vi "Move to final location.vi"(8 "error in (no error)":errorcluster, 11 "DAQOrcaFlash in":refnum<class "DAQOrcaFlash.lvclass">) -> (0 "error out":errorcluster, 3 "DAQOrcaFlash out":refnum<class "DAQOrcaFlash.lvclass">)   [LabVIEW 2012, in "DAQOrcaFlash.lvclass"]
uses:
  DAQOrcaFlash.lvclass
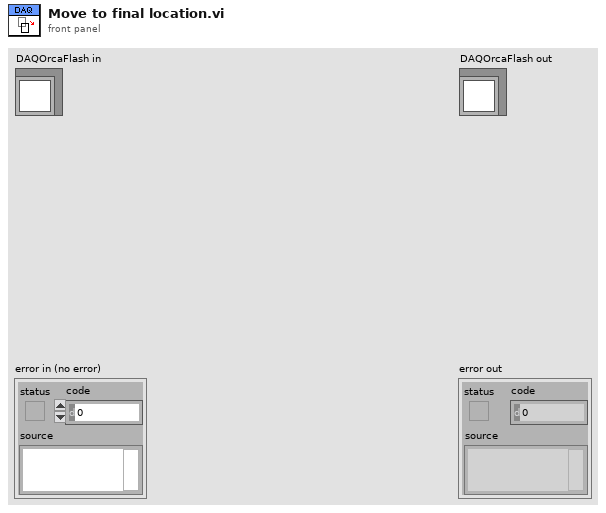
[diagram p1: front panel]
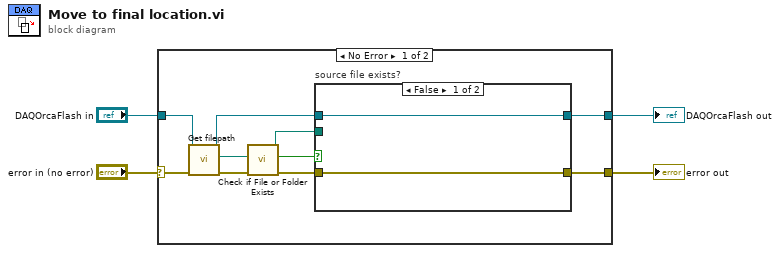
[diagram p0: block diagram]
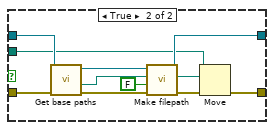
[diagram p2: hidden frame]
diagram:
  n1 = case shown="No Error" "error in (no error)" {
    selector: "error in (no error)" -> [w14 w29]
    tunnel: [w13 w29] -> w3
    tunnel: [w10 w28] -> w1
    tunnel: "DAQOrcaFlash in" -> [w11 w28]
    frame No Error {
      n2 = call "Get filepath.vi"("error in (no error)"=w14, "DAQOrcaFlash in"=w11) -> ("error out"=w7:errorcluster, "full storage path"=w9:path, "DAQOrcaFlash out"=w12:refnum<class "DAQOrcaFlash.lvclass">)  [unwired: 7 in]
      n3 = call <vilib>:"Check if File or Folder Exists.vi"("error in (no error)"=w7, "path"=w9) -> ("error out"=w6:errorcluster, "file or folder exists?"=w5:bool, "dup path"=w8:path)  [unwired: 7 in]
      n4 = case "source file exists?" shown="False" w5 {
        tunnel: [w15 w25] -> w13
        tunnel: w12 -> [w16 w24]
        tunnel: [w16 w22] -> w10
        tunnel: w8 -> [_ w18]
        tunnel: w6 -> [w15 w17]
        frame False {
        }
        frame True {
          n5 = call-dynamic "Get base paths.vi"("error in (no error)"=w17, "DAQOrcaFlash in"=w24) -> ("error out"=w27:errorcluster, "final conversion folder"=w21:path, "DAQOrcaFlash out"=w23:refnum<class "DAQOrcaFlash.lvclass">)  [unwired: 6 in, 1 out]
          n6 = call "Make filepath.vi"("error in (no error)"=w27, "is cxd file path?"=FALSE, "base path"=w21, "DAQOrcaFlash in"=w23) -> ("error out"=w26:errorcluster, "filepath out"=w19:path, "DAQOrcaFlash out"=w22:refnum<class "DAQOrcaFlash.lvclass">)  [unwired: 5 in]
          n7 = Move(source path=w18, error in=w26, 10:w19) -> (error out=w25:errorcluster)  [unwired: 2 in, 2 out]
        }
      }
    }
    frame Error {
    }
  }
  "error out" <- w3
  "DAQOrcaFlash out" <- w1
